vi "Display Timeout Popup.vi"(6 "Theme":refnum<class "Theme.lvclass">, 8 "error in":errorcluster, 9 "Timeout (s)":dbl=1.0 min=1.0, 10 "Message":string, 11 "Graphic":T1="info") -> (0 "error out":errorcluster, 2 "Timeout":bool)   [LabVIEW 2021, in "Pop-Up.lvlib" / "Timeout.lvclass"]
doc: "The timeout popup will display information to the user and wait the specified timeout depending on the number of seconds passed into this VI.\n\n<b>Note:</b> The function <b>Close Pop-Up.vi</b> can be used to close this dialog early.\n\nInputs:\n-Graphic [typedef combobox] - Image (PNG) for Graphic for Popup\n-Message [String] - String Variable to populate Display\n-Theme [lvclass] - the theme for the style of the popup\n-Timeout (s) [DBL] - the amount of seconds for the timeout\n\n<b>Code Developed By:</b>\nDaniel Coons\nTechnology Service Corporation\n1983 S Liberty Drive\nBloomington, IN 47403\nPhone: 812 558-7100\ndaniel.coons@tsc.com\nwww.tsc.com/atcs"
uses:
  Timeout.lvclass
  Graphics.ctl
  Theme/Theme.lvclass
  C:/Development/Open Source/tsc-pop-up/Popup/Popup.lvclass
  Timeout.lvclass/Timeout.ctl
  Popup/Popup.lvclass/Popup.ctl
  Popup/Popup.lvclass
  Pop-Up.lvlib
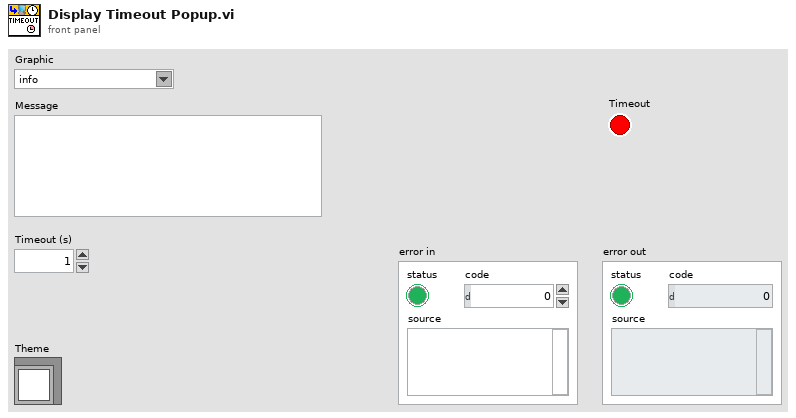
[diagram p1: front panel]
types:
  T1 = typedef "Pop-Up.lvlib/Graphics.ctl" = string
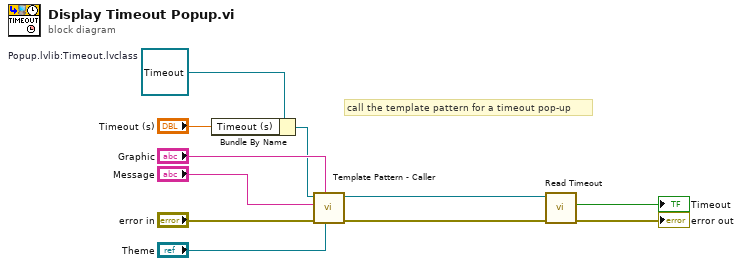
[diagram p0: block diagram]
diagram:
  w5 = refnum<class "Timeout.lvclass"> refnum  # Popup.lvlib:Timeout.lvclass
  # "call the template pattern for a timeout pop-up"
  n1 = Bundle By Name(cluster=w5, "Timeout (s)"="Timeout (s)") -> (w4:refnum<class "Timeout.lvclass">)
  n2 = call-dynamic "Template Pattern - Caller.vi"("Theme"="Theme", "standard"="Graphic", "error in (no error)"="error in", "Message"="Message", "Pop-Up in"=w4) -> ("error out"=w10:errorcluster, "Pop-Up out"=w2:refnum<class "Timeout.lvclass">)  [unwired: 5 in]
  n3 = call "Read Timeout.vi"("error in (no error)"=w10, "Popup in"=w2) -> ("error out"=→"error out":errorcluster, "Timeout?"=→"Timeout":bool)  [unwired: 7 in, 1 out]
